vi "Close Frame.vi"(8 "error in (no error)":errorcluster, 9 "timeout ms (5000)":i32=5000, 11 "WebSockets in":refnum<class "WebSocket.lvclass">) -> (0 "error out":errorcluster, 3 "WebSockets out":refnum<class "WebSocket.lvclass">)   [LabVIEW 2013, in "WebSockets.lvlib" / "WebSocket.lvclass"]
doc: "Sends a WebSocket close frame to the connection endpoint but does not close the underlying socket connection."
uses:
  WebSocket.lvclass
  Opcodes.ctl
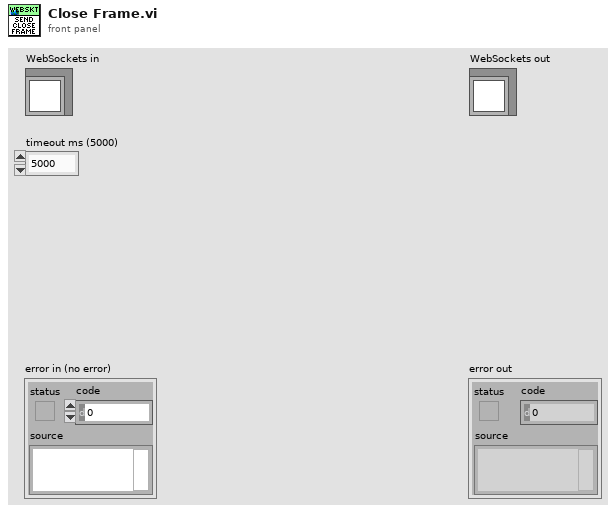
[diagram p1: front panel]
types:
  T1 = typedef "WebSockets.lvlib/WebSocket.lvclass/Opcodes.ctl" = u8
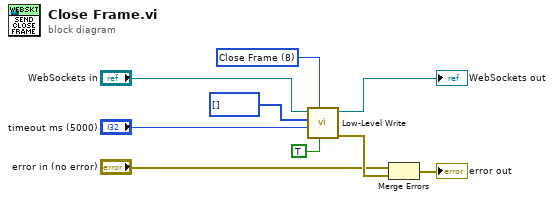
[diagram p0: block diagram]
diagram:
  w5 = T1 8 items=["Cont. Frame"=0, "Text"=1, "Binary"=2, "Close Frame"=8, "Ping"=9, "Pong"=10] ("Opcode (Text)")
  n1 = call "Low-Level Write.vi"("Mask payload?"=TRUE, "Opcode (Text)"=w5, "timeout ms (5000)"="timeout ms (5000)", "Data"=u8[] [], "WebSockets in"="WebSockets in") -> ("error out"=w9:errorcluster, "WebSockets out"=→"WebSockets out":refnum<class "WebSocket.lvclass">)  [unwired: 5 in]
  n2 = Merge Errors("error in (no error)", w9) -> (→"error out":errorcluster)
